vi "GetFixtureSerialNumber.vi"(0 "Sequence Path":path=path "C:/ModisEdge/Scope/Test Sequence/Modis Edge Scope Test.seq", 1 "name or relative path":string="ModisEdge.ini", 3 "error in (no error)":errorcluster) -> (6 "Fixture Serial Number":string="2015-433-0002-1", 7 "OK":bool=TRUE, 9 "error out":errorcluster)   [LabVIEW 2015]
uses:
  <vilib>/Utility/config.llb/Read Key (String).vi
  <vilib>/Utility/config.llb/Write Key (String).vi
  <vilib>/Utility/config.llb/NI_LVConfig.lvlib
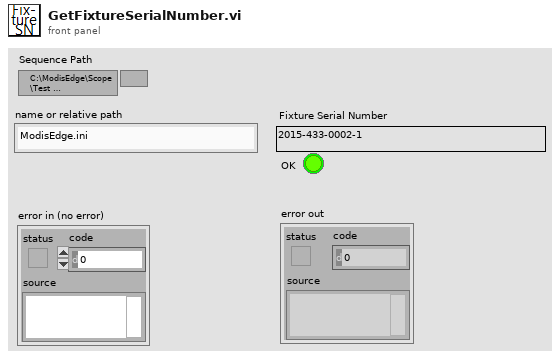
[diagram p1: front panel]
types:
  T1 = typedef "NI_LVConfig.lvlib/Config Data RefNum.ctl" = refnum<k1>
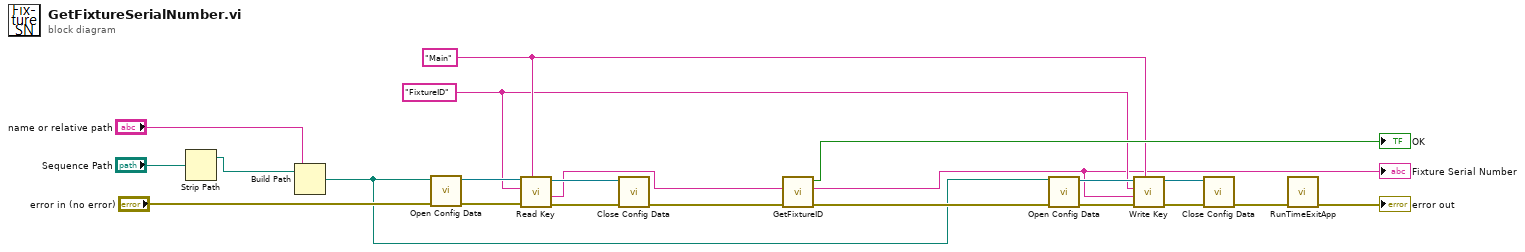
[diagram p0: block diagram]
diagram:
  w10 = "Main" ("section")
  w9 = "FixtureID" ("key")
  n1 = Strip Path(path="Sequence Path") -> (stripped path=w3:path)  [unwired: 1 out]
  n2 = Build Path(base path=w3, name or relative path="name or relative path") -> (appended path=w7:path)
  n3 = call <vilib>:"Open Config Data.vi"("error in (no error)"="error in (no error)", "configuration file path"=w7) -> ("error out"=w16:errorcluster, "refnum"=w19:T1)  [unwired: 7 in, 1 out]
  n4 = call-poly <vilib>:"Read Key.vi"("section"=w10, "error in (no error)"=w16, "key"=w9, "refnum"=w19) -> ("error out"=w17:errorcluster, "value"=w2:string, "refnum out"=w18:T1)  [unwired: 4 in, 1 out]
  n5 = call <vilib>:"Close Config Data.vi"("error in (no error)"=w17, "refnum"=w18) -> ("error out"=w20:errorcluster)  [unwired: 8 in, 1 out]
  n6 = call "GetFixtureID.vi"("error in (no error)"=w20, "String"=w2) -> ("error out"=w11:errorcluster, "Fixture Serial Number"=w1:string, "OK"=→"OK":bool)  [unwired: 7 in]
  "Fixture Serial Number" <- w1
  n7 = call <vilib>:"Open Config Data.vi"("error in (no error)"=w11, "configuration file path"=w7) -> ("error out"=w14:errorcluster, "refnum"=w13:T1)  [unwired: 7 in, 1 out]
  n8 = call-poly <vilib>:"Write Key.vi"("section"=w10, "error in (no error)"=w14, "value"=w1, "key"=w9, "refnum"=w13) -> ("error out"=w15:errorcluster, "refnum out"=w12:T1)  [unwired: 4 in, 1 out]
  n9 = call <vilib>:"Close Config Data.vi"("error in (no error)"=w15, "refnum"=w12) -> ("error out"=w6:errorcluster)  [unwired: 8 in, 1 out]
  n10 = call "RunTimeExitApp.vi"("error in (no error)"=w6) -> ("error out"=→"error out":errorcluster)  [unwired: 10 in]
